vi "NF WF1973_74 QUES Ntr.vi"(6 "Read(F)":bool, 8 "error in (no error)":errorcluster caption="Error IN", 10 "Q_NTR(0)":i32(knob) min=0 max=65535 step=1 scale=0.0..65535.0, 11 "VISAsession":refnum<visa-resource-name>) -> (0 "error out":errorcluster caption="Error OUT", 2 "Query Q_NTR":i32=99999, 3 "CopyVISAsession":refnum<visa-resource-name>)   [LabVIEW 2010]
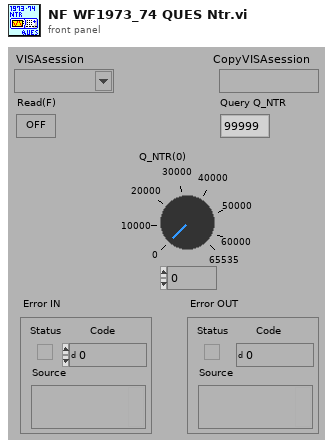
[diagram p1: front panel]
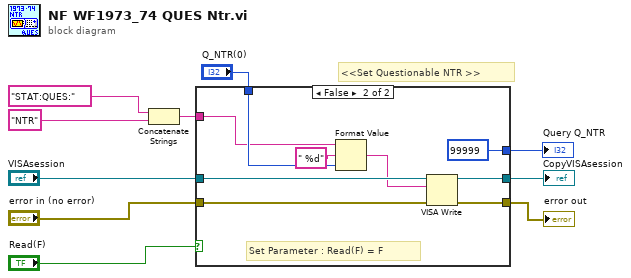
[diagram p0: block diagram]
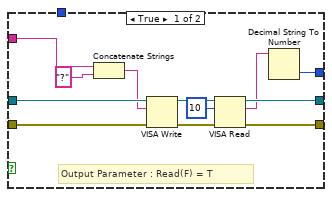
[diagram p2: hidden frame]
diagram:
  # "<<Set Questionable NTR >>"
  n1 = Concatenate Strings("STAT:QUES:" ("文字列"), "NTR" ("文字列")) -> (w3:string)
  n2 = case shown="FALSE" "Read(F)" {
    tunnel: "VISAsession" -> [w22 w31]
    tunnel: [w13 w28] -> w9
    tunnel: [w19 w29] -> w8
    tunnel: "error in (no error)" -> [w18 w30]
    tunnel: w3 -> [w16 w24]
    tunnel: "Q_NTR(0)" -> [_ w25]
    tunnel: [w11 99999] -> w4
    frame True {
      # "Output Parameter : Read(F) = T"
      n3 = Concatenate Strings(w16, "?" ("形式文字列")) -> (w14:string)
      n4 = VISA Write(VISA resource name=w22, write buffer=w14, error in (no error)=w18) -> (VISA resource name out=w20:refnum<visa-resource-name>, error out=w21:errorcluster)  [unwired: 1 out]
      n5 = VISA Read(VISA resource name=w20, byte count=u32 10 ("バイトカウント（0）"), error in (no error)=w21) -> (VISA resource name out=w13:refnum<visa-resource-name>, read buffer=w12:string, error out=w19:errorcluster)  [unwired: 1 out]
      n6 = Decimal String To Number(string=w12) -> (number=w11:i32)  [unwired: 2 in, 1 out]
    }
    frame False {
      # "Set Parameter : Read(F) = F"
      n7 = Format Value(string ("")=w24, format string=" %d" ("形式文字列"), value (0)=w25) -> (output string=w23:string)
      n8 = VISA Write(VISA resource name=w31, write buffer=w23, error in (no error)=w30) -> (VISA resource name out=w28:refnum<visa-resource-name>, error out=w29:errorcluster)  [unwired: 1 out]
    }
  }
  "error out" <- w8
  "CopyVISAsession" <- w9
  "Query Q_NTR" <- w4
